vi "44xx AI Min and Max.vi"(9 "AI.channels":tag, 10 "446x AI":T2) -> (1 "DAQ Type":T1, 2 "AI.Max":dbl, 3 "AI.Min":dbl)   [LabVIEW 2016, in "Lockin.DAQ.lvclass"]
uses:
  Lockin.DAQ.lvclass
  Typedefs/446xAI-enum.ctl
  Typedefs/DAQType-enum.ctl
  <resource>/objmgr/daqmx.rc
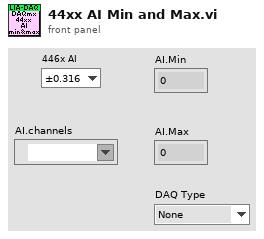
[diagram p1: front panel]
types:
  T1 = typedef "Lockin.DAQ.lvclass/DAQType-enum.ctl" = enum16{"None", "USB 4431", "PXI 446x"}
  T2 = typedef "Lockin.DAQ.lvclass/446xAI-enum.ctl" = enum16{"±0.316", "±1.00", "±3.16", "±10.0", "±31.6", "±42.4"}
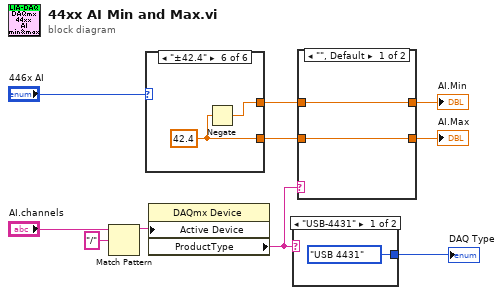
[diagram p0: block diagram]
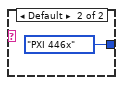
[diagram p2: hidden frame]
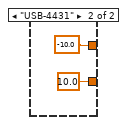
[diagram p3: hidden frame]
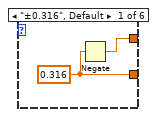
[diagram p4: hidden frame]
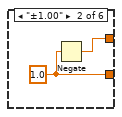
[diagram p5: hidden frame]
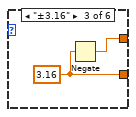
[diagram p6: hidden frame]
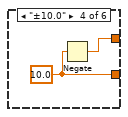
[diagram p7: hidden frame]
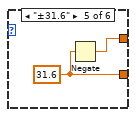
[diagram p8: hidden frame]
diagram:
  n1 = Match Pattern(string="AI.channels", regular expression="/") -> (before substring=w8:string)  [unwired: 1 in, 3 out]
  n2 = case shown="\"±42.4\"" "446x AI" {
    tunnel: [w11 w13 w15 w17 w19 w21] -> w5
    tunnel: [w12 w14 w16 w18 w20 w22] -> w3
    frame "±0.316", Default {
      w12 = 0.316 ("AI.Min")
      n3 = Negate(x=w12) -> (-x=w11:dbl)
    }
    frame "±1.00" {
      w14 = 1.0 ("AI.Min")
      n4 = Negate(x=w14) -> (-x=w13:dbl)
    }
    frame "±3.16" {
      w16 = 3.16 ("AI.Min")
      n5 = Negate(x=w16) -> (-x=w15:dbl)
    }
    frame "±10.0" {
      w18 = 10.0 ("AI.Min")
      n6 = Negate(x=w18) -> (-x=w17:dbl)
    }
    frame "±31.6" {
      w20 = 31.6 ("AI.Min")
      n7 = Negate(x=w20) -> (-x=w19:dbl)
    }
    frame "±42.4" {
      w22 = 42.4 ("AI.Min")
      n8 = Negate(x=w22) -> (-x=w21:dbl)
    }
  }
  n9 = property class="DAQmx Device"("Active Device"=w8) -> ("ProductType"=w2:string)  [unwired: 2 in, 2 out]
  n10 = case shown="\"USB-4431\"" w2 {
    tunnel: [DAQType-enum."USB 4431" ("DAQ Type") DAQType-enum."PXI 446x" ("DAQ Type")] -> w1
    frame "USB-4431" {
    }
    frame Default {
    }
  }
  "DAQ Type" <- w1
  n11 = case shown="\"\", Default" w2 {
    tunnel: [w26 -10.0] -> w6
    tunnel: w5 -> [w26 _]
    tunnel: [w25 10.0 ("AI.Min")] -> w4
    tunnel: w3 -> [w25 _]
    frame "", Default {
    }
    frame "USB-4431" {
    }
  }
  "AI.Min" <- w6
  "AI.Max" <- w4
